vi "Constants.vi"() -> ()   [LabVIEW 2020, in "Regatron G5 Custom Device Shared.lvlib"]
doc: "Use this Global VI to access the GUIDs assigned to the page resources of the Custom Device."
uses:
  Regatron G5 Custom Device Shared.lvlib
panel:
  in  "Tab Control":enum32{"GUIDs", "Constants", "Properties"}(tab)
  in  "Regatron G5 Custom Device":string="8d66f1c2-52ba-458c-a1c0-de3f11fce76b"
  in  "IP Address":string="Compiled.Settings"
  in  "Compiled.Settings":string="Compiled.Settings"
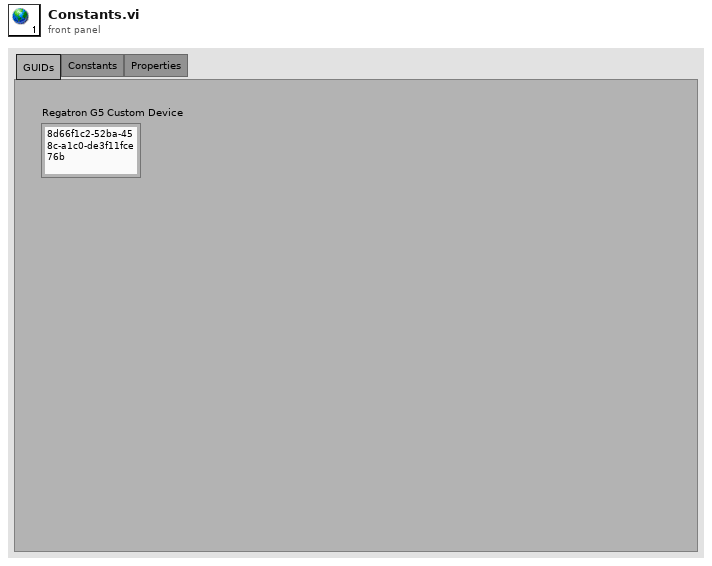
[diagram p1: front panel]
diagram:
